vi "NI VeriStand - Connect to System.vi"(4 "Filtered Targets":string[](array[string]), 6 "Deploy System Definition (T)":bool=TRUE, 7 "Calibration File":path, 8 "error in (no error)":errorcluster, 9 "Timeout (60000 ms)":u32=60000, 10 "System Definition File (.nivssdf)":path, 11 "WorkspaceManager in":T1) -> (0 "error out":errorcluster, 3 "WorkspaceManager out":T1)   [LabVIEW 2020, in "NI_VS Workspace ExecutionAPI.lvlib"]
doc: "Connects the VeriStand Gateway to the target(s) you define in the system definition file you specify."
uses:
  <vilib>/NI VeriStand/Execution/Workspace/NI_VS Workspace ExecutionAPI.lvlib
  <vilib>/NI VeriStand/Execution/Workspace/WorkspaceAPI.ctl
  NationalInstruments.VeriStand.ClientAPI
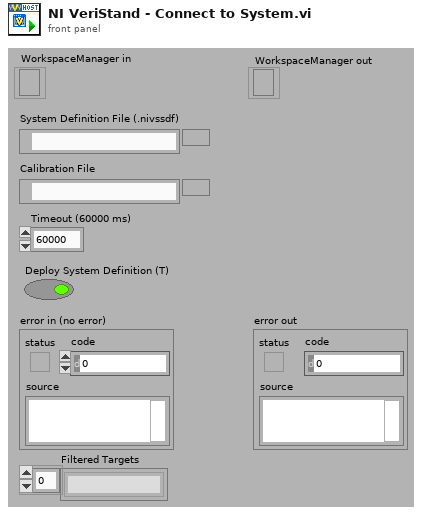
[diagram p1: front panel]
types:
  T1 = typedef "NI_VS Workspace ExecutionAPI.lvlib/WorkspaceAPI.ctl" = refnum<k24>
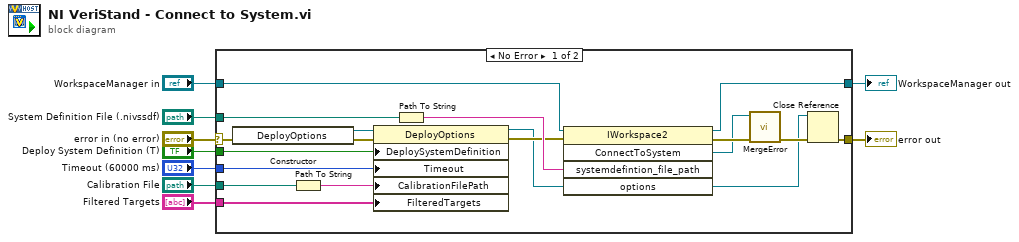
[diagram p0: block diagram]
diagram:
  n1 = case shown="No Error" "error in (no error)" {
    selector: "error in (no error)" -> [w16 w29]
    tunnel: "WorkspaceManager in" -> [w26 w28]
    tunnel: "System Definition File (.nivssdf)" -> [w25 _]
    tunnel: [w23 w28] -> w7
    tunnel: "Calibration File" -> [w20 _]
    tunnel: "Deploy System Definition (T)" -> [w19 _]
    tunnel: "Timeout (60000 ms)" -> [w18 _]
    tunnel: [w12 w29] -> w2
    tunnel: "Filtered Targets" -> [w10 _]
    frame No Error {
      n2 = constructor class="DeployOptions"(error in=w16) -> (reference out=w21:refnum<k24>, error out=w15:errorcluster)  [unwired: 2 in, 1 out]
      n3 = Path To String(path=w20) -> (string=w17:string)
      n4 = property class="DeployOptions"(reference=w21, error in=w15, "DeploySystemDefinition"=w19, "Timeout"=w18, "CalibrationFilePath"=w17, "FilteredTargets"=w10) -> (reference out=w11:refnum<k24>, error out=w14:errorcluster)
      n5 = Path To String(path=w25) -> (string=w24:string)
      n6 = invoke class="IWorkspace2" method="ConnectToSystem"(reference=w26, error in=w14, "systemdefintion_file_path"=w24, "options"=w11) -> (reference out=w23:T1, error out=w27:errorcluster, "ConnectToSystem"=w22:refnum<k24>)  [unwired: 1 in, 2 out]
      n7 = call <vilib>:"MergeError.vi"("error in (no error)"=w27, "Error"=w22) -> ("error out"=w13:errorcluster)  [unwired: 9 out]
      n8 = Close Reference(reference=w11, error in (no error)=w13) -> (error out=w12:errorcluster)
    }
    frame Error {
    }
  }
  "WorkspaceManager out" <- w7
  "error out" <- w2
